vi "export_VI.vi"() -> ()   [LabVIEW 2020]
uses:
  <vilib>/Utility/file.llb/Write Delimited Spreadsheet (string).vi
panel:
  in  "y":bool
  out "Filtered Pahse":dbl[](graph)
  out "Raw Phase":dbl[](graph)
  in  "file path (dialog if empty)":path
  out "Amplitude":dbl[](graph)
  out "output cluster":T1
  in  "Detail of the export csv":T1
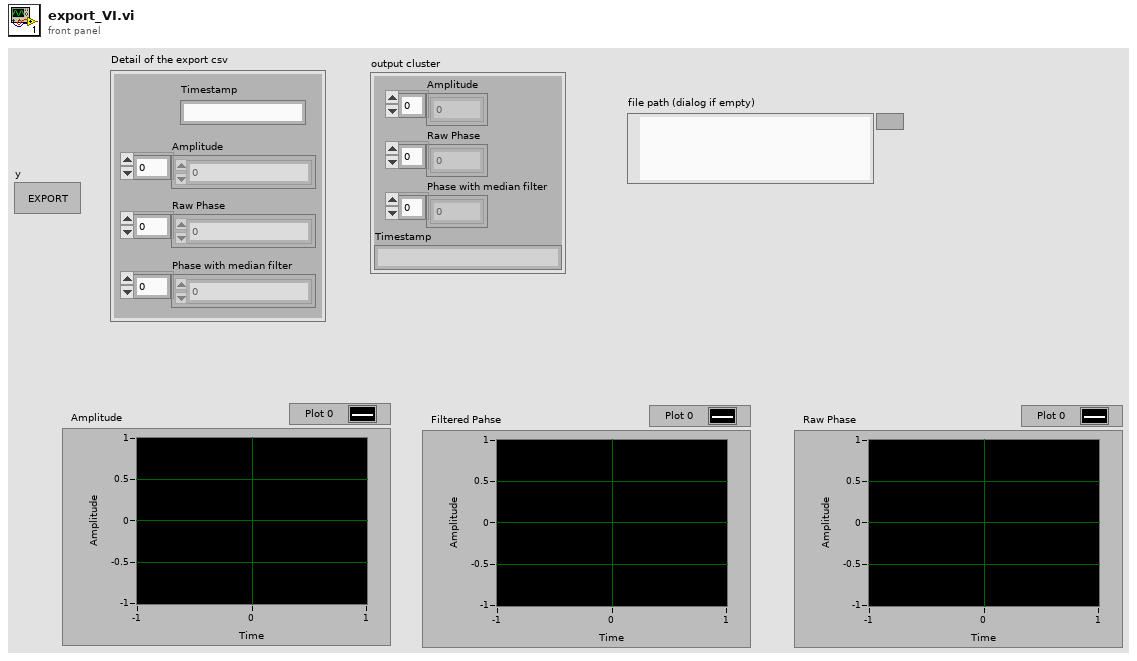
[diagram p1: front panel]
types:
  T1 = cluster{"Amplitude":dbl[], "Raw Phase":dbl[], "Phase with median filter":dbl[], "Timestamp":string}
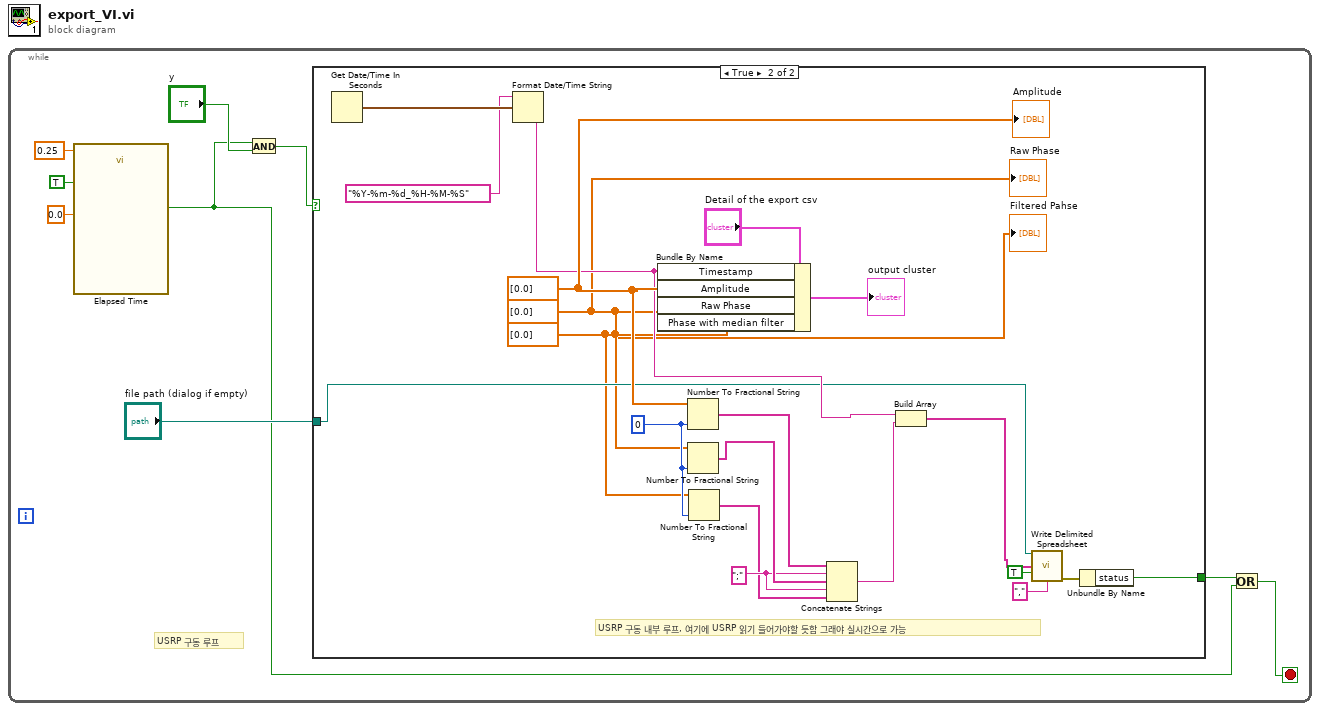
[diagram p0: block diagram]
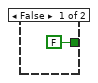
[diagram p2: hidden frame]
diagram:
  n1 = while {
    stop <- w1 stop-if-true
    # "USRP 구동 루프"
    n2 = call "Elapsed Time"("Time Target (s)"=0.25, "Auto Reset"=TRUE, "Set Start Time (s)"=0.0) -> ("Time has Elapsed"=w2:bool)  [unwired: 9 in, 7 out]
    n3 = And(x=w2, y="y") -> (x .and. y?=w5:bool)
    n4 = case shown="True" w5 {
      tunnel: "file path (dialog if empty)" -> [_ w16]
      tunnel: [FALSE ("status") w12] -> w3
      frame False {
      }
      frame True {
        w23 = ";"
        w26 = i16 0 ("precision (6)")
        w14 = dbl[] [0.0] ("Phase with median filter")
        w15 = dbl[] [0.0] ("Raw Phase")
        w27 = dbl[] [0.0] ("Amplitude")
        # "USRP 구동 내부 루프, 여기에 USRP 읽기 들어가야할 듯함 그래야 실시간으로 가능"
        n5 = Get Date/Time In Seconds() -> (seconds since 1Jan1904=w30:timestamp)
        n6 = Format Date/Time String(time format string (%c)="%Y-%m-%d_%H-%M-%S", seconds (now)=w30) -> (date/time string=w20:string)  [unwired: 1 in]
        n7 = Bundle By Name(cluster="Detail of the export csv", "Timestamp"=w20, "Amplitude"=w27, "Raw Phase"=w15, "Phase with median filter"=w14) -> (→"output cluster":T1)
        n8 = Number To Fractional String(number=w27, precision (6)=w26) -> (F-format string=w25:string[])  [unwired: 2 in]
        n9 = Number To Fractional String(number=w15, precision (6)=w26) -> (F-format string=w24:string[])  [unwired: 2 in]
        n10 = Number To Fractional String(number=w14, precision (6)=w26) -> (F-format string=w22:string[])  [unwired: 2 in]
        n11 = Concatenate Strings(w25, w23, w24, w23, w22) -> (w21:string)
        n12 = Build Array(w20, w21) -> (w17:string[])
        n13 = call-poly <vilib>:"Write Delimited Spreadsheet.vi"("file path (dialog if empty)"=w16, "1D data"=w17, "append to file? (new file:F)"=TRUE, "delimiter (\\t)"="," ("delimiter (\\t)")) -> ("error out"=w13:errorcluster)  [unwired: 10 in, 1 out]
        n14 = Unbundle By Name "Unbundle By Name"(w13) -> ("status"=w12:bool)
        "Amplitude" <- w27
        "Raw Phase" <- w15
        "Filtered Pahse" <- w14
      }
    }
    n15 = Or(x=w3, y=w2) -> (x .or. y?=w1:bool)
  }
